vi "Save Batt Data(2).vi"(6 "Error In":errorcluster, 9 "Battery Capture":u64) -> (0 "error out":errorcluster, 2 "Pass/Fail #":i32, 3 "Pass?":bool)   [LabVIEW 2013]
uses:
  <vilib>/Utility/NIReport.llb/NI_report.lvclass
  <vilib>/Utility/NIReport.llb/Excel/NI_Excel.lvclass
  <vilib>/addons/_office/NI_ReportGenerationToolkit.lvlib
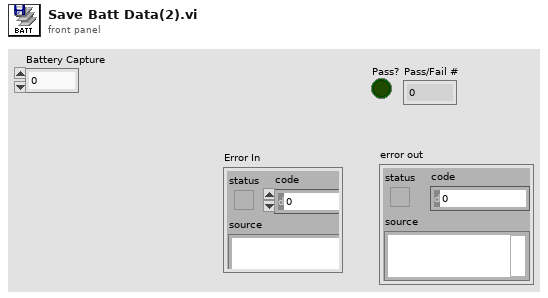
[diagram p1: front panel]
types:
  T1 = enum16{"maximized", "minimized", "normal", "no change"}
  T2 = enum16{"Standard Report", "HTML", "Word", "Excel"}
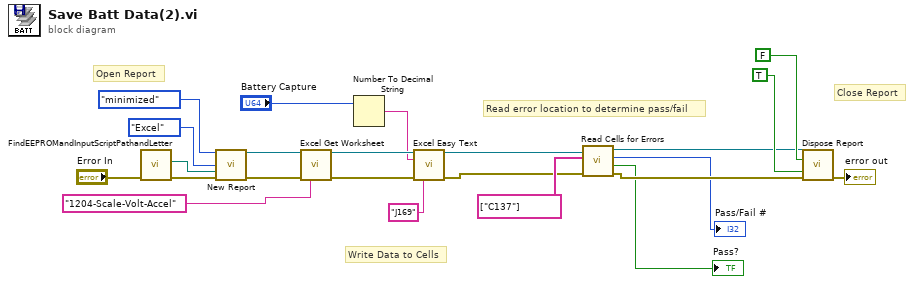
[diagram p0: block diagram]
diagram:
  # "Open Report"
  # "Close Report"
  # "Read error location to determine pass/fail"
  # "Write Data to Cells"
  n1 = call "FindEEPROMandInputScriptPathandLetter.vi"("Error In"="Error In") -> ("Error Out"=w14:errorcluster, "Engr Result Path"=w18:path)  [unwired: 6 in, 1 out]
  n2 = call <vilib>:"New Report.vi"("window state (normal)"=T1."minimized", "report type"=T2."Excel", "template (empty)"=w18, "error in (no error)"=w14) -> ("report out"=w16:refnum<class "NI_report.lvclass">, "error out"=w17:errorcluster)  [unwired: 10 in]
  n3 = call <vilib>:"Excel Get Worksheet.vi"("report in"=w16, "error in (no error)"=w17, "name (\"\")"="1204-Scale-Volt-Accel" ("name (\"\")")) -> ("report out"=w12:refnum<class "NI_report.lvclass">, "error out"=w11:errorcluster)  [unwired: 11 in]
  n4 = Number To Decimal String(number="Battery Capture") -> (decimal integer string=w1:string)  [unwired: 1 in]
  n5 = call <vilib>:"Excel Easy Text.vi"("report in"=w12, "text"=w1, "error in (no error)"=w11, "name (\"\")"="J169") -> ("report out"=w10:refnum<class "NI_report.lvclass">, "error out"=w8:errorcluster)  [unwired: 7 in, 3 out]
  n6 = call "Read Cells for Errors.vi"("error in (no error)"=w8, "Error Cells (ex:A12)"=string[] ["C137"] ("Array"), "NI_report in"=w10) -> ("error out"=w6:errorcluster, "Pass?"=→"Pass?":bool, "Error Code"=→"Pass/Fail #":i32, "NI_report out"=w7:refnum<class "NI_report.lvclass">)  [unwired: 5 in]
  n7 = call-dynamic "Dispose Report.vi"("report in"=w7, "wait until printing completed? (T)"=FALSE, "save changes? (F)"=TRUE, "error in (no error)"=w6) -> ("error out"=→"error out":errorcluster)  [unwired: 11 in]
